vi "RSToutput.vi"(6 "RST Motor Constants":T1={"Pitch Gain (2*pi/enc)"=1.0, "Output Sign"=[1.0, -1.0, 1.0], "Phase Offset (rad)"=0.0, "Saturation"=32000.0}, 9 "Encoder Position":dbl, 11 "Command":dbl) -> (1 "Coerced?":bool, 3 "Control":dbl[](array[numeric]))   [LabVIEW 2011, in "kevLib2011.lvlib"]
uses:
  kevLib2011.lvlib
  RSTtypeDef.ctl
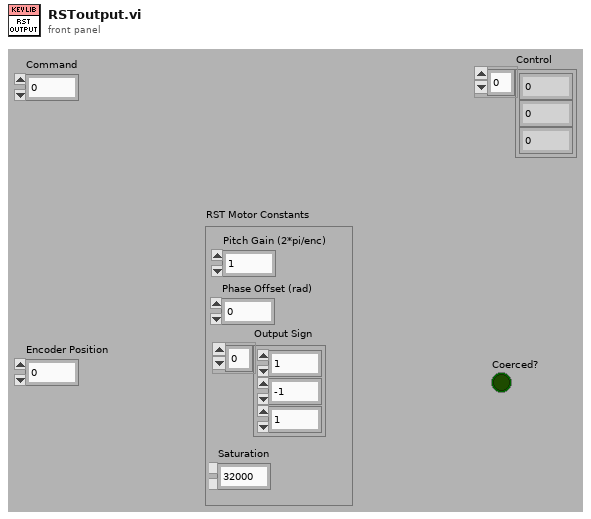
[diagram p1: front panel]
types:
  T1 = typedef "kevLib2011.lvlib/RSTtypeDef.ctl" = cluster{"Pitch Gain (2*pi/enc)":dbl, "Output Sign":dbl[], "Phase Offset (rad)":dbl, "Saturation":dbl}
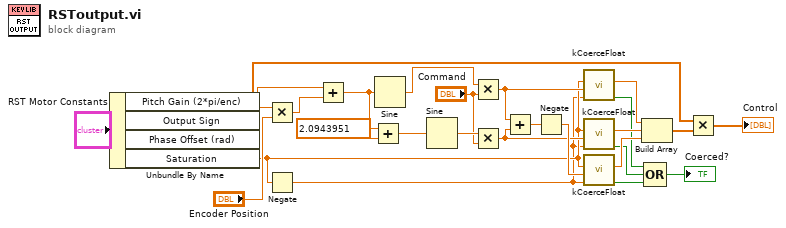
[diagram p0: block diagram]
diagram:
  n1 = Unbundle By Name("RST Motor Constants") -> ("Pitch Gain (2*pi/enc)"=w25:dbl, "Output Sign"=w1:dbl[], "Phase Offset (rad)"=w23:dbl, "Saturation"=w8:dbl)
  n2 = Multiply(x=w25, y="Encoder Position") -> (x*y=w24:dbl)
  n3 = Negate(x=w8) -> (-x=w7:dbl)
  n4 = Add(x=w23, y=w24) -> (x+y=w6:dbl)
  n5 = Add(x=2.0943951, y=w6) -> (x+y=w5:dbl)
  n6 = Sine(x=w6) -> (sin(x)=w22:dbl)
  n7 = Sine(x=w5) -> (sin(x)=w21:dbl)
  n8 = Multiply(x=w22, y="Command") -> (x*y=w18:dbl)
  n9 = Multiply(x=w21, y="Command") -> (x*y=w16:dbl)
  n10 = Add(x=w18, y=w16) -> (x+y=w19:dbl)
  n11 = Negate(x=w19) -> (-x=w17:dbl)
  n12 = call "kCoerceFloat.vi"("lower"=w7, "input"=w18, "upper"=w8) -> ("coerced?"=w12:bool, "output"=w15:dbl)  [unwired: 7 in]
  n13 = call "kCoerceFloat.vi"("lower"=w7, "input"=w16, "upper"=w8) -> ("coerced?"=w11:bool, "output"=w14:dbl)  [unwired: 7 in]
  n14 = call "kCoerceFloat.vi"("lower"=w7, "input"=w17, "upper"=w8) -> ("coerced?"=w10:bool, "output"=w13:dbl)  [unwired: 7 in]
  n15 = Build Array(w15, w14, w13) -> (w3:dbl[])
  n16 = Compound Arithmetic op=OR(w12, w11, w10) -> (→"Coerced?":bool)
  n17 = Multiply(x=w1, y=w3) -> (x*y=→"Control":dbl[])
